vi "Ex2_LabVIEW_bartelmj.vi"() -> ()   [LabVIEW 2016]
panel:
  out "X":dbl
  out "Y":dbl
  in  "N":dbl
  in  "y":dbl
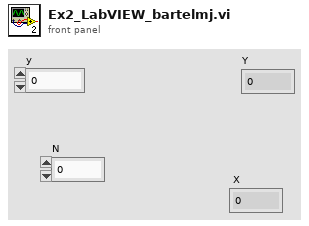
[diagram p1: front panel]
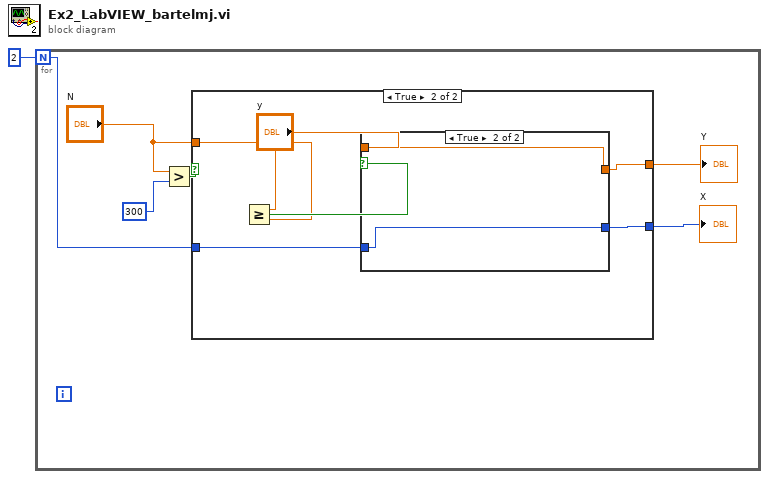
[diagram p0: block diagram]
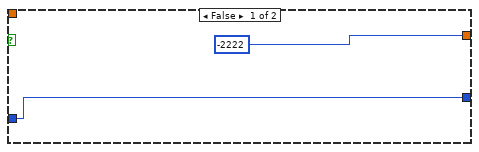
[diagram p2: hidden frame]
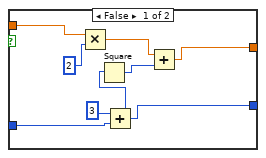
[diagram p3: hidden frame]
diagram:
  n1 = for {
    N: 2 -> [w3]
    n2 = Greater?(x="N", y=300) -> (0:w6:bool)
    n3 = case shown="True" w6 {
      tunnel: [-2222 w13] -> w4
      tunnel: "N" -> [_ w12]
      tunnel: w3 -> [w8 w11]
      tunnel: [w8 w10] -> w2
      frame False {
      }
      frame True {
        n4 = Greater Or Equal?(x="y", y=w12) -> (x >= y?=w15:bool)
        n5 = case shown="True" w15 {
          tunnel: "y" -> [w22 w25]
          tunnel: [w19 w25] -> w13
          tunnel: w11 -> [w17 w24]
          tunnel: [w16 w24] -> w10
          frame False {
            n6 = Multiply(x=w22, y=2) -> (x*y=w21:dbl)
            n7 = Add(x=3, y=w17) -> (x+y=w16:i32)
            n8 = Square(x=w16) -> (x^2=w23:i32)
            n9 = Add(x=w21, y=w23) -> (x+y=w19:dbl)
          }
          frame True {
          }
        }
      }
    }
    "Y" <- w4
    "X" <- w2
  }
